vi "PathPlanner_CommandUtil_Execute.vi"(11 "Command":T1) -> ()   [LabVIEW 2019, in "PathPlanner24.lvlib"]
doc: "Issues the given command.\n\nCurrently the only type of commands that can be issued are Boolean commands. The value is forced to TRUE when the command is issued.\n\nThe following table lists the actions performed for different types of commands:\n - Unknown - nothing - not supported.\n - Wait - nothing - not supported\n - Named - Issue boolean command with TRUE value using the \"name\" as the command name.\n - Path - nothing - not supported\n - Sequential, Parallel, Race, Deadline - Issue boolean command with TRUE value for each of the commands contained in the \"commands\" array. The value for \"name\" is used as the command name.\n\nInputs:\n -- Command - cluster - Command definition.\n\nOutputs:\n -- <none>"
uses:
  PathPlanner24.lvlib
  TypeDef/PathPlannerCommandUtil.ctl
  ENum/PathPlanner_CommandUtilType_ENUM.ctl
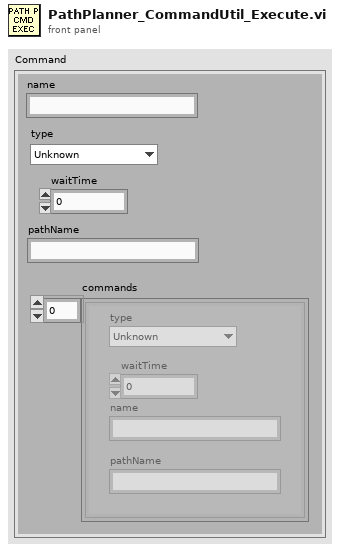
[diagram p1: front panel]
types:
  T1 = typedef "PathPlanner24.lvlib/PathPlannerCommandUtil.ctl" = cluster{"waitTime":dbl, "name":string, "pathName":string, "commands":cluster{"type":T2, "waitTime":dbl, "name":string, "pathName":string}[], "type":T2}
  T2 = typedef "PathPlanner24.lvlib/PathPlanner_CommandUtilType_ENUM.ctl" = enum16{"Unknown", "Wait", "Named", "Path", "Sequential", "Parallel", "Race", "Deadline"}
  T3 = cluster{"type":T2, "waitTime":dbl, "name":string, "pathName":string}[]
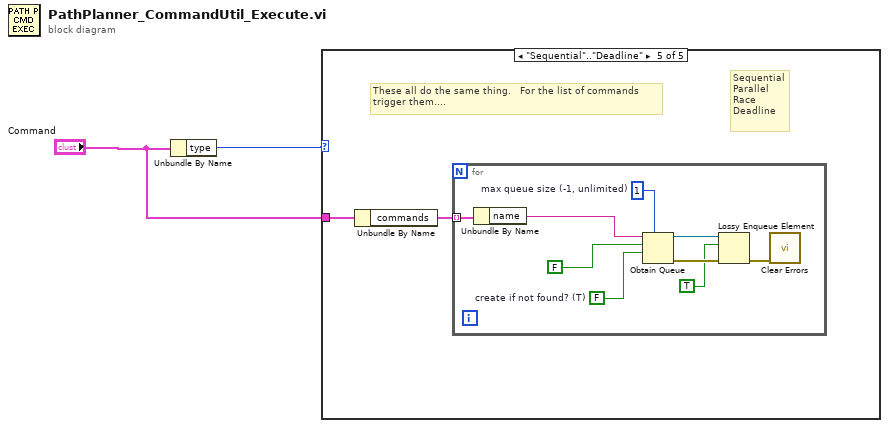
[diagram p0: block diagram]
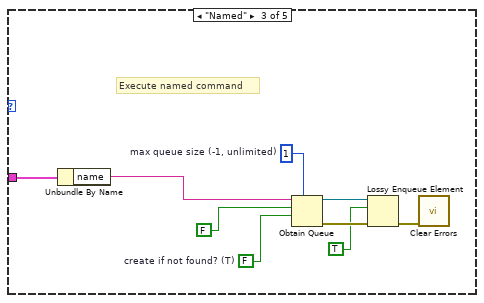
[diagram p4: hidden frame]
diagram:
  n1 = Unbundle By Name("Command") -> ("type"=w2:T2)
  n2 = case shown="\"Sequential\"..\"Deadline\"" w2 {
    tunnel: "Command" -> [_ _ w11 _ w13]
    frame "Unknown" {
      # "Unknown -- do nothiing"
    }
    frame "Wait" {
      # "Wait - do nothing..."
    }
    frame "Named" {
      w5 = FALSE  # create if not found? (T)
      w4 = 1  # max queue size (-1, unlimited)
      # "Execute named command"
      n3 = Unbundle By Name(w11) -> ("name"=w3:string)
      n4 = Obtain Queue(max queue size (-1, unlimited)=w4, name (unnamed)=w3, element data type=FALSE, create if not found? (T)=w5) -> (queue out=w8:refnum<queue>, error out=w9:errorcluster)  [unwired: 1 in, 1 out]
      n5 = Lossy Enqueue Element(queue=w8, element=TRUE, error in (no error)=w9) -> (error out=w10:errorcluster)  [unwired: 3 out]
      n6 = call <vilib>:"Clear Errors.vi"("error in (no error)"=w10) -> ()  [unwired: 5 in, 2 out]
    }
    frame "Path" {
      # "Do nothing.....  for now..."
    }
    frame "Sequential".."Deadline" {
      # "Sequential\nParallel\nRace\nDeadline"
      # "These all do the same thing.   For the list of commands\ntrigger them...."
      n7 = Unbundle By Name(w13) -> ("commands"=w12:T3)
      n8 = for {
        tunnel: w12 -> [w22] mode=indexing
        w20 = FALSE  # create if not found? (T)
        w21 = 1  # max queue size (-1, unlimited)
        n9 = Unbundle By Name(w22) -> ("name"=w14:string)
        n10 = Obtain Queue(max queue size (-1, unlimited)=w21, name (unnamed)=w14, element data type=FALSE, create if not found? (T)=w20) -> (queue out=w18:refnum<queue>, error out=w17:errorcluster)  [unwired: 1 in, 1 out]
        n11 = Lossy Enqueue Element(queue=w18, element=TRUE, error in (no error)=w17) -> (error out=w15:errorcluster)  [unwired: 3 out]
        n12 = call <vilib>:"Clear Errors.vi"("error in (no error)"=w15) -> ()  [unwired: 5 in, 2 out]
      }
    }
  }
